vi "IsPreviousReady.vi"(8 "wait for":T2, 9 "Active slaves":T2={"camera"=TRUE, "Tektronik"=TRUE, "Motors"=FALSE, "Gage"=FALSE}, 10 "element":T3) -> (2 "is ready":bool)   [LabVIEW 2018, in "MasterProgramSupportFunctions.lvlib"]
uses:
  MasterProgramSupportFunctions.lvlib
  NetworkStream/NetworkStreamData.ctl
  ActiveSlaves.ctl
  MasterStatus.ctl
  NetworkStream/NetworkStream.lvlib
  MySharedVariables.lvlib
panel:
  out "MasterStatusShared":T1
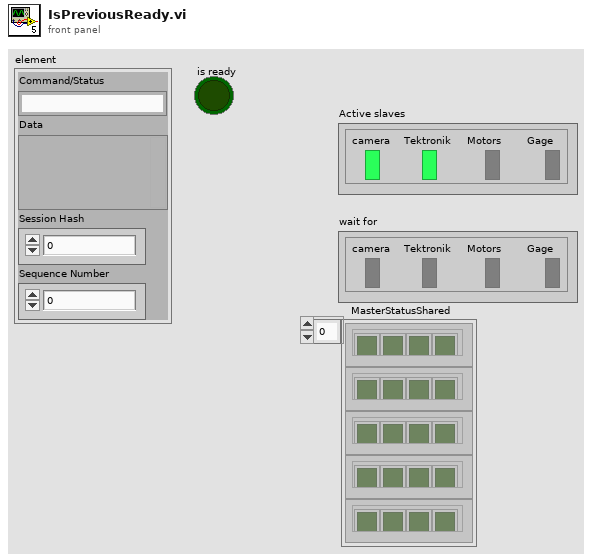
[diagram p1: front panel]
types:
  T1 = typedef "MySharedVariables.lvlib/MasterStatus.ctl" = cluster{"Camera done":bool, "Tektronik done":bool, "Motors done":bool, "Gage done":bool}[]
  T2 = typedef "MasterProgramSupportFunctions.lvlib/ActiveSlaves.ctl" = cluster{"camera":bool, "Tektronik":bool, "Motors":bool, "Gage":bool}
  T3 = typedef "NetworkStream.lvlib/NetworkStreamData.ctl" = cluster{"Command/Status":string, "Data":variant, "Session Hash":u64, "Sequence Number":u64}
  T4 = cluster{"Camera done":bool, "Tektronik done":bool, "Motors done":bool, "Gage done":bool}
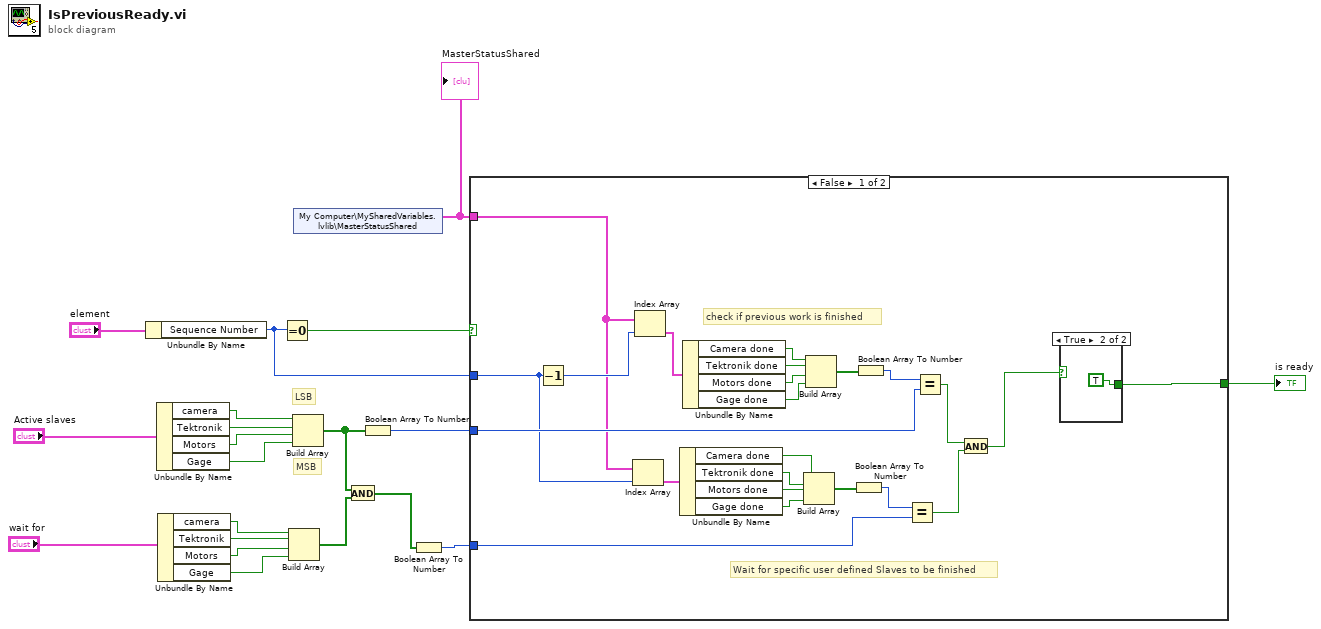
[diagram p0: block diagram]
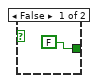
[diagram p2: hidden frame]
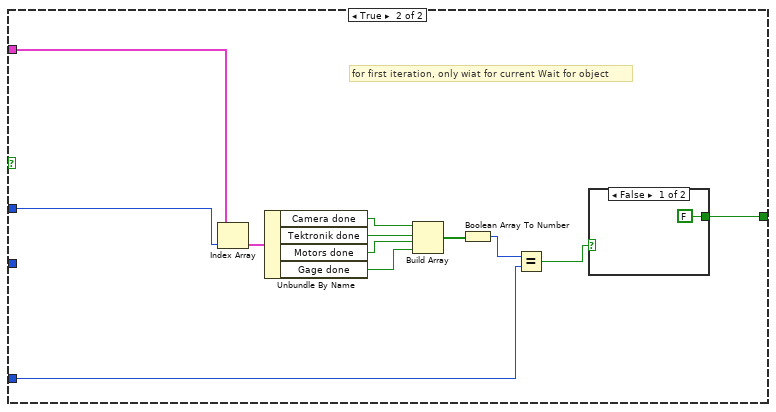
[diagram p3: hidden frame]
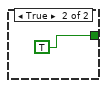
[diagram p4: hidden frame]
diagram:
  # "MSB"
  # "LSB"
  n1 = Unbundle By Name("element") -> ("Sequence Number"=w17:u64)
  n2 = Unbundle By Name("Active slaves") -> ("camera"=w16:bool, "Tektronik"=w15:bool, "Motors"=w14:bool, "Gage"=w13:bool)
  n3 = Unbundle By Name("wait for") -> ("camera"=w11:bool, "Tektronik"=w10:bool, "Motors"=w9:bool, "Gage"=w8:bool)
  n4 = Equal To 0?(x=w17) -> (x = 0?=w18:bool)
  n5 = Build Array(w11, w10, w9, w8) -> (w4:bool[])
  n6 = Build Array(w16, w15, w14, w13) -> (w5:bool[])
  n7 = shared-variable "My Computer\\MySharedVariables.lvlib\\MasterStatusShared"() -> (w6:T1)  [unwired: 1 in, 1 out]
  "MasterStatusShared" <- w6
  n8 = And(x=w5, y=w4) -> (x .and. y?=w3:bool[])
  n9 = Boolean Array To Number(Boolean array=w5) -> (number=w12:u32)
  n10 = Boolean Array To Number(Boolean array=w3) -> (number=w7:u32)
  n11 = case shown="False" w18 {
    tunnel: [w43 w46] -> w19
    tunnel: w17 -> [w33 w57]
    tunnel: w12 -> [w34 _]
    tunnel: w7 -> [w25 w48]
    tunnel: w6 -> [w21 w56]
    frame False {
      # "Wait for specific user defined Slaves to be finished"
      # "check if previous work is finished"
      n12 = Decrement(x=w33) -> (x-1=w42:u64)
      n13 = Index Array(array=w21, index=w33) -> (element=w32:T4)
      n14 = Index Array(array=w21, index=w42) -> (element=w41:T4)
      n15 = Unbundle By Name(w32) -> ("Camera done"=w31:bool, "Tektronik done"=w30:bool, "Motors done"=w29:bool, "Gage done"=w28:bool)
      n16 = Unbundle By Name(w41) -> ("Camera done"=w40:bool, "Tektronik done"=w39:bool, "Motors done"=w38:bool, "Gage done"=w37:bool)
      n17 = Build Array(w31, w30, w29, w28) -> (w27:bool[])
      n18 = Build Array(w40, w39, w38, w37) -> (w36:bool[])
      n19 = Boolean Array To Number(Boolean array=w27) -> (number=w26:u32)
      n20 = Boolean Array To Number(Boolean array=w36) -> (number=w35:u32)
      n21 = Equal?(x=w26, y=w25) -> (x = y?=w23:bool)
      n22 = Equal?(x=w35, y=w34) -> (x = y?=w24:bool)
      n23 = And(x=w24, y=w23) -> (x .and. y?=w22:bool)
      n24 = case shown="True" w22 {
        tunnel: [FALSE ("is ready") TRUE ("is ready")] -> w43
        frame False {
        }
        frame True {
        }
      }
    }
    frame True {
      # "for first iteration, only wiat for current Wait for object"
      n25 = Index Array(array=w56, index=w57) -> (element=w55:T4)
      n26 = Unbundle By Name(w55) -> ("Camera done"=w54:bool, "Tektronik done"=w53:bool, "Motors done"=w52:bool, "Gage done"=w51:bool)
      n27 = Build Array(w54, w53, w52, w51) -> (w50:bool[])
      n28 = Boolean Array To Number(Boolean array=w50) -> (number=w49:u32)
      n29 = Equal?(x=w49, y=w48) -> (x = y?=w47:bool)
      n30 = case shown="False" w47 {
        tunnel: [FALSE ("is ready") TRUE ("is ready")] -> w46
        frame False {
        }
        frame True {
        }
      }
    }
  }
  "is ready" <- w19
